vi "Upload.vi"(7 "ICAN":refnum<class "ICAN.lvclass">, 8 "Error In":errorcluster, 9 "Multiplexer":cluster{"Index":u16, "Sub-Index":u8} {"Index" format="%.0x"}, 10 "Node-ID":u8, 11 "reference in":refnum<class "SDO Manager.lvclass">) -> (0 "Error Out":errorcluster, 1 "Value":u8[](array[numeric]) format="%.0x", 2 "Success?":bool, 3 "reference out":refnum<class "SDO Manager.lvclass">)   [LabVIEW 2024, in "CANopen Master.lvlib" / "SDO Manager.lvclass"]
uses:
  SDO Manager.lvclass
  HAL/HAL/Protocols/ICAN/ICAN.lvclass
  CANopen Message/CANopen Message.lvclass/CANopen Message.ctl
  CANopen Message/CANopen Message.lvclass
  SDO Manager.lvclass/SDO Manager.ctl
  Service Data Object/Service Data Object.lvclass
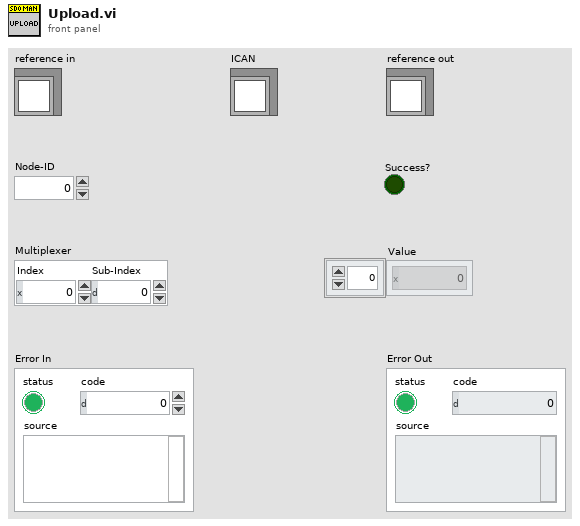
[diagram p1: front panel]
types:
  T1 = typedef "CANopen Master.lvlib/SDO Manager.lvclass/ObjectAttributes.ctl" = cluster{"SDO Response Map":map{u32, refnum<notifier>}}
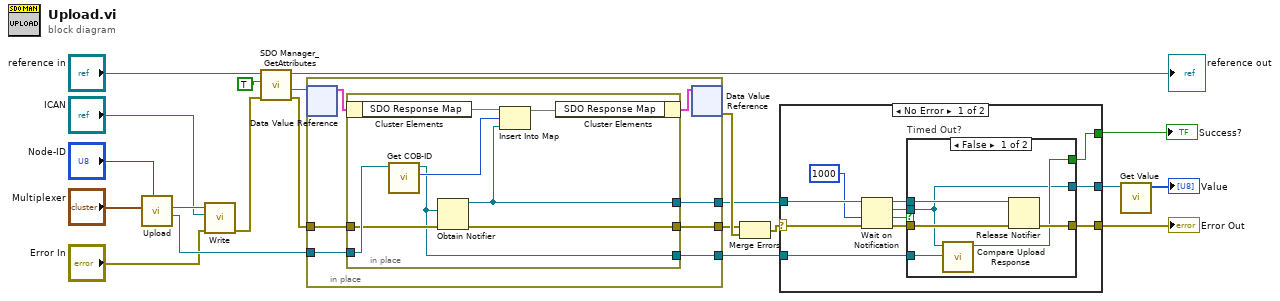
[diagram p0: block diagram]
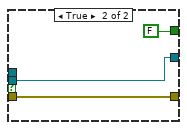
[diagram p2: hidden frame]
diagram:
  n1 = call "Upload.vi"("Node-ID"="Node-ID", "Multiplexer"="Multiplexer") -> ("CANopen Response Message"=w12:refnum<class "CANopen Message.lvclass">, "CANopen Message out"=w18:refnum<class "CANopen Message.lvclass">)  [unwired: 7 in, 1 out]
  n2 = call "Write.vi"("error in"="Error In", "ICAN"="ICAN", "CANopen Message in"=w18) -> ("error out"=w14:errorcluster)  [unwired: 7 in, 1 out]
  n3 = call "SDO Manager_GetAttributes.vi"("Error In"=w14, "OnlyGetDvrReference(False)"=TRUE, "reference in"="reference in") -> ("Error Out"=w6:errorcluster, "DataRef"=w13:refnum<data-value>, "reference out"=→"reference out":refnum<class "SDO Manager.lvclass">)  [unwired: 5 in, 1 out]
  n4 = in-place {
    in-place-border: w12 -> [w27]
    in-place-border: [w26] -> w10
    in-place-border: [w25] -> w8
    in-place-border: w6 -> [w24]
    in-place-border: [w22] -> w3
    n5 = in-place-dvr #1(w13) -> (w28:T1)  [unwired: 1 out]
    n6 = in-place {
      in-place-border: w27 -> [w32]
      in-place-border: [w33] -> w26
      in-place-border: [w31] -> w25
      in-place-border: w24 -> [w30]
      in-place-border: [w29] -> w22
      n7 = in-place-cluster #2(w28) -> ("SDO Response Map"=w36:map{u32, refnum<notifier>})
      n8 = call "Get COB-ID.vi"("CANopen Message in"=w32) -> ("COB-ID"=w34:u32, "CANopen Message out"=w29:refnum<class "CANopen Message.lvclass">)  [unwired: 9 in]
      n9 = Obtain Notifier(notification data type=w29, error in (no error)=w30) -> (notifier out=w31:refnum<notifier>, error out=w33:errorcluster)  [unwired: 2 in, 1 out]
      n10 = Insert Into Map(map in=w36, key=w34, value=w31) -> (map out=w35:map{u32, refnum<notifier>})  [unwired: 2 out]
      n11 = in-place-cluster #2("SDO Response Map"=w35) -> (w23:T1)
    }
    n12 = in-place-dvr #1(w23) -> (w11:errorcluster)  [unwired: 1 out]
  }
  n13 = Merge Errors(w10, w11) -> (w9:errorcluster)
  n14 = case shown="No Error" w9 {
    selector: w9 -> [w45 w57]
    tunnel: w8 -> [w47 _]
    tunnel: [w43 w57] -> w7
    tunnel: [w38 _] -> w5
    tunnel: [w37 _] -> w2
    tunnel: w3 -> [w40 _]
    frame No Error {
      n15 = Wait on Notification(notifier=w47, timeout in ms (-1)=1000, error in (no error)=w45) -> (notifier out=w42:refnum<notifier>, notification=w41:refnum<class "CANopen Message.lvclass">, timed out?=w39:bool, error out=w44:errorcluster)  [unwired: 1 in]
      n16 = case "Timed Out?" shown="False" w39 {
        tunnel: w44 -> [w53 w56]
        tunnel: [w52 w56] -> w43
        tunnel: w42 -> [w51 _]
        tunnel: w41 -> [w48 w55]
        tunnel: w40 -> [w50 _]
        tunnel: [w49 FALSE ("Equal?")] -> w38
        tunnel: [w48 w55] -> w37
        frame False {
          n17 = call "Compare Upload Response.vi"("Expected"=w50, "Actual"=w48) -> ("Equal?"=w49:bool)  [unwired: 9 in]
          n18 = Release Notifier(notifier=w51, error in (no error)=w53) -> (error out=w52:errorcluster)  [unwired: 1 in, 2 out]
        }
        frame True {
        }
      }
    }
    frame Error {
    }
  }
  "Error Out" <- w7
  "Success?" <- w5
  n19 = call "Get Value.vi"("CANopen Message"=w2) -> ("Value"=→"Value":u8[])  [unwired: 10 in]
